vi "start watchdog schedule.vi"(7 "comms queue":refnum<queue>, 10 "comms in":T1, 11 "message scheduler in":refnum<class "message scheduler.lvclass">) -> (3 "comms out":T1)   [LabVIEW 2018]
uses:
  Chris VIs/Message Scheduler/message scheduler.lvclass
  type defs/comms loop data.ctl
  Chris VIs/Incident logger/Incident logger.lvclass
  <vilib>/Modbus/master/Modbus Master.lvclass
  Chris VIs/Message Scheduler/generic message queue/standard message queue/standard message.lvclass
  D:/Chris/oneDrive/OneDrive - Imperial College London/LabVIEW/Chris VIs/Message Scheduler/generic message queue/generic message.lvclass
  Chris VIs/Message Scheduler/scheduled message/scheduled message.lvclass
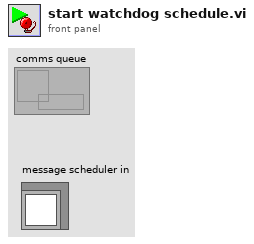
[diagram p1: front panel]
types:
  T1 = typedef "comms loop data.ctl" = cluster{"params":cluster{"commandStream":cluster{"reader name":string, "writer name":string, "stream buffer size":i32}, "errorStream":cluster{"reader name":string, "writer name":string, "stream buffer size":i32}, "RT IP address":string, "pulserControllerIP":string}, "vars":cluster{"commandStream":refnum<k21>, "Incident logger":refnum<class "Incident logger.lvclass">, "check error scheduled message":u32, "errorStream":refnum<k21>, "watchdogScheduleID":u32, "pulsator":cluster{"pulser connection":refnum<class "Modbus Master.lvclass">, "pulserConnected":bool, "pulsatorScheduleID":u32, "pulserRunning":bool}}}
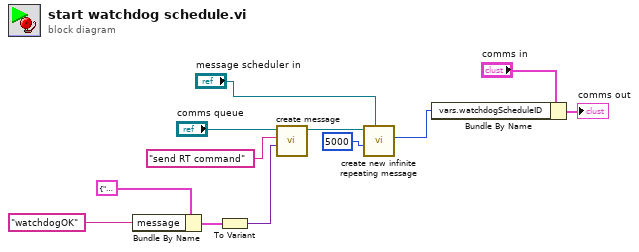
[diagram p0: block diagram]
diagram:
  n1 = Bundle By Name(cluster=cluster{"message":string, "data":variant} {"message"="", "data"=variant} ("element"), "message"="watchdogOK") -> (w4:cluster{"message":string, "data":variant})
  n2 = To Variant(anything=w4) -> (Variant=w3:variant)
  n3 = call "create message.vi"("data"=w3, "message"="send RT command", "queue ref"="comms queue") -> ("standard message out"=w8:refnum<class "standard message.lvclass">)  [unwired: 7 in, 1 out]
  n4 = call "create new infinite repeating message.vi"("message scheduler"="message scheduler in", "ms delay"=u32 5000, "message"=w8) -> ("schedule ID"=w11:u32)  [unwired: 7 in, 1 out]
  n5 = Bundle By Name(cluster="comms in", "vars.watchdogScheduleID"=w11) -> (→"comms out":T1)
